vi "add channel to TEC configuration.vi"(8 "error in":errorcluster, 10 "channel":refnum<class "TBM channel.lvclass">, 11 "TEC configuration in":refnum<class "TEC configuration.lvclass">) -> (0 "error out":errorcluster, 3 "TEC configuration out":refnum<class "TEC configuration.lvclass">)   [LabVIEW 2013, in "TEC configuration.lvclass"]
uses:
  TEC configuration.lvclass
  <vilib>/NI/Tag Bus Module Framework/channel/TBM channel.lvclass
  TEC configuration.lvclass/TEC configuration.ctl
  <vilib>/NI/Tag Bus/tag/tag descriptor.lvclass/tag descriptor.ctl
  <vilib>/NI/Tag Bus/tag/tag descriptor.lvclass
  <vilib>/NI/Configuration Framework/NISE_CEF_TreeControl.lvlib
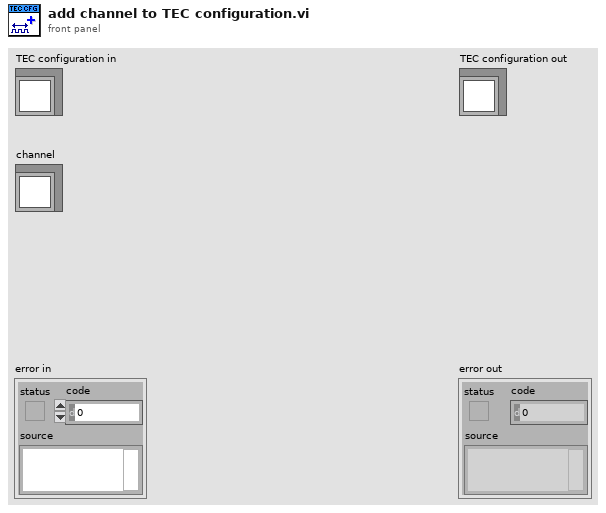
[diagram p1: front panel]
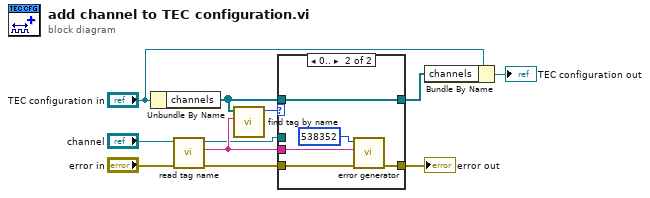
[diagram p0: block diagram]
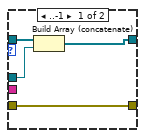
[diagram p2: hidden frame]
diagram:
  n1 = Unbundle By Name("TEC configuration in") -> ("channels"=w3:refnum<class "TBM channel.lvclass">[])
  n2 = call <vilib>:"read tag name.vi"("error in"="error in", "system tag in"="channel") -> ("error out"=w6:errorcluster, "name"=w4:string, "system tag out"=w2:refnum<class "TBM channel.lvclass">)  [unwired: 7 in]
  n3 = call <vilib>:"find tag by name.vi"("name"=w4, "tags in"=w3) -> ("index"=w7:i32)  [unwired: 9 in]
  n4 = case shown="0.." w7 {
    tunnel: w6 -> [w12 w19]
    tunnel: [w12 w18] -> w5
    tunnel: w4 -> [_ w17]
    tunnel: w3 -> [w15 w16]
    tunnel: w2 -> [w14 _]
    tunnel: [w13 w16] -> w1
    frame ..-1 {
      n5 = Build Array (concatenate)(w15, w14) -> (w13:refnum<class "TBM channel.lvclass">[])
    }
    frame 0.. {
      n6 = call <vilib>:"error generator.vi"("error in"=w19, "append error message"=w17, "error code (0)"=538352) -> ("error out"=w18:errorcluster)  [unwired: 6 in]
    }
  }
  "error out" <- w5
  n7 = Bundle By Name(cluster="TEC configuration in", "channels"=w1) -> (→"TEC configuration out":refnum<class "TEC configuration.lvclass">)
